vi "Find Index.vi"(0 "Array":bool[](array[boolean])) -> (4 "Index":string)   [LabVIEW 2024]
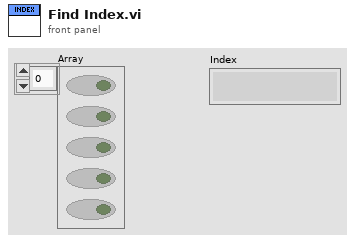
[diagram p1: front panel]
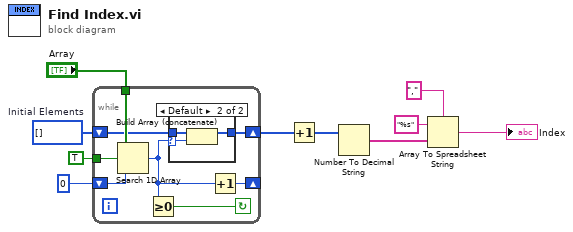
[diagram p0: block diagram]
diagram:
  w9 = i32[] []  # Initial Elements
  n1 = while {
    shift-right: [w11] -> _
    shift-left: 0 -> [w18]
    shift-right: [w15] -> w3
    shift-left: w9 -> [w16]
    tunnel: "Array" -> [w17]
    tunnel: TRUE ("Element Data") -> [w14]
    stop <- w12 continue-if-true
    n2 = Search 1D Array(1D array=w17, element=w14, start index (0)=w18) -> (index of element=w13:i32)
    n3 = Greater Or Equal To 0?(x=w13) -> (x >= 0?=w12:bool)
    n4 = case shown="Default" w13 {
      selector: w13 -> [_ w22]
      tunnel: w16 -> [w19 w21]
      tunnel: [w19 w20] -> w15
      frame -1 {
      }
      frame Default {
        n5 = Build Array (concatenate)(w21, w22) -> (w20:i32[])
      }
    }
    n6 = Increment(x=w13) -> (x+1=w11:i32)
  }
  n7 = Increment(x=w3) -> (x+1=w1:i32[])
  n8 = Number To Decimal String(number=w1) -> (decimal integer string=w2:string[])  [unwired: 1 in]
  n9 = Array To Spreadsheet String(delimiter (Tab)=",", array=w2, 3:"%s" ("format string")) -> (spreadsheet string=→"Index":string)
